vi "Measurement Logic.vi"() -> ()   [LabVIEW 2024, in "NIDmmDCRmsVoltage.lvlib"]
uses:
  NIDmmDCRmsVoltage.lvlib
  <vilib>/MeasurementLink/MeasurementLink Measurement Server/Measure Call Context/Measure Call Context.lvclass
  Typedefs/Measurement Result.ctl
  Typedefs/Measurement Configuration.ctl
  Typedefs/Function.ctl
  Typedefs/Resolution Digits.ctl
  <instrlib>/niDMM/nidmm.llb/niDMM Resolution in Digits.ctl
  <instrlib>/niDMM/nidmm.llb/niDMM Read Waveform (waveform data).vi
  <vilib>/measure/madcrms.llb/Basic Averaged DC-RMS for 1 Chan.vi
  <vilib>/MeasurementLink/MeasurementLink Session Management V1/Session Reservation/Session Reservation.lvclass
  <vilib>/MeasurementLink/MeasurementLink niDMM/MeasurementLink niDMM.lvlib
  <vilib>/MeasurementLink/MeasurementLink niDMM/Initialize Sessions - 1Sess.vi
  <instrlib>/niDMM/nidmm.llb/niDMM Configure Measurement Digits.vi
  <vilib>/measure/NI_MAPro.lvlib
panel:
  in  "measurement configuration":T1={"Range"=10.0, "Function"=1003, "Resolution in Digits"=enum."5 1/2", "Number of Samples"=2000.0, "Pin Name"="", "Sample Rate (Hz)"=20000.0} {"Function" items=["Waveform_Voltage"=1003, "Waveform_Current"=1004]}
  out "Waveform Graph 2":waveform(dbl)(graph)
  in  "Instrument Descriptor":refnum<k15>="DMM1"
  in  "error in":errorcluster
  out "error out":errorcluster
  out "measurement results":T4
  out "measure call context out":refnum<class "Measure Call Context.lvclass">
  in  "measure call context in":refnum<class "Measure Call Context.lvclass">
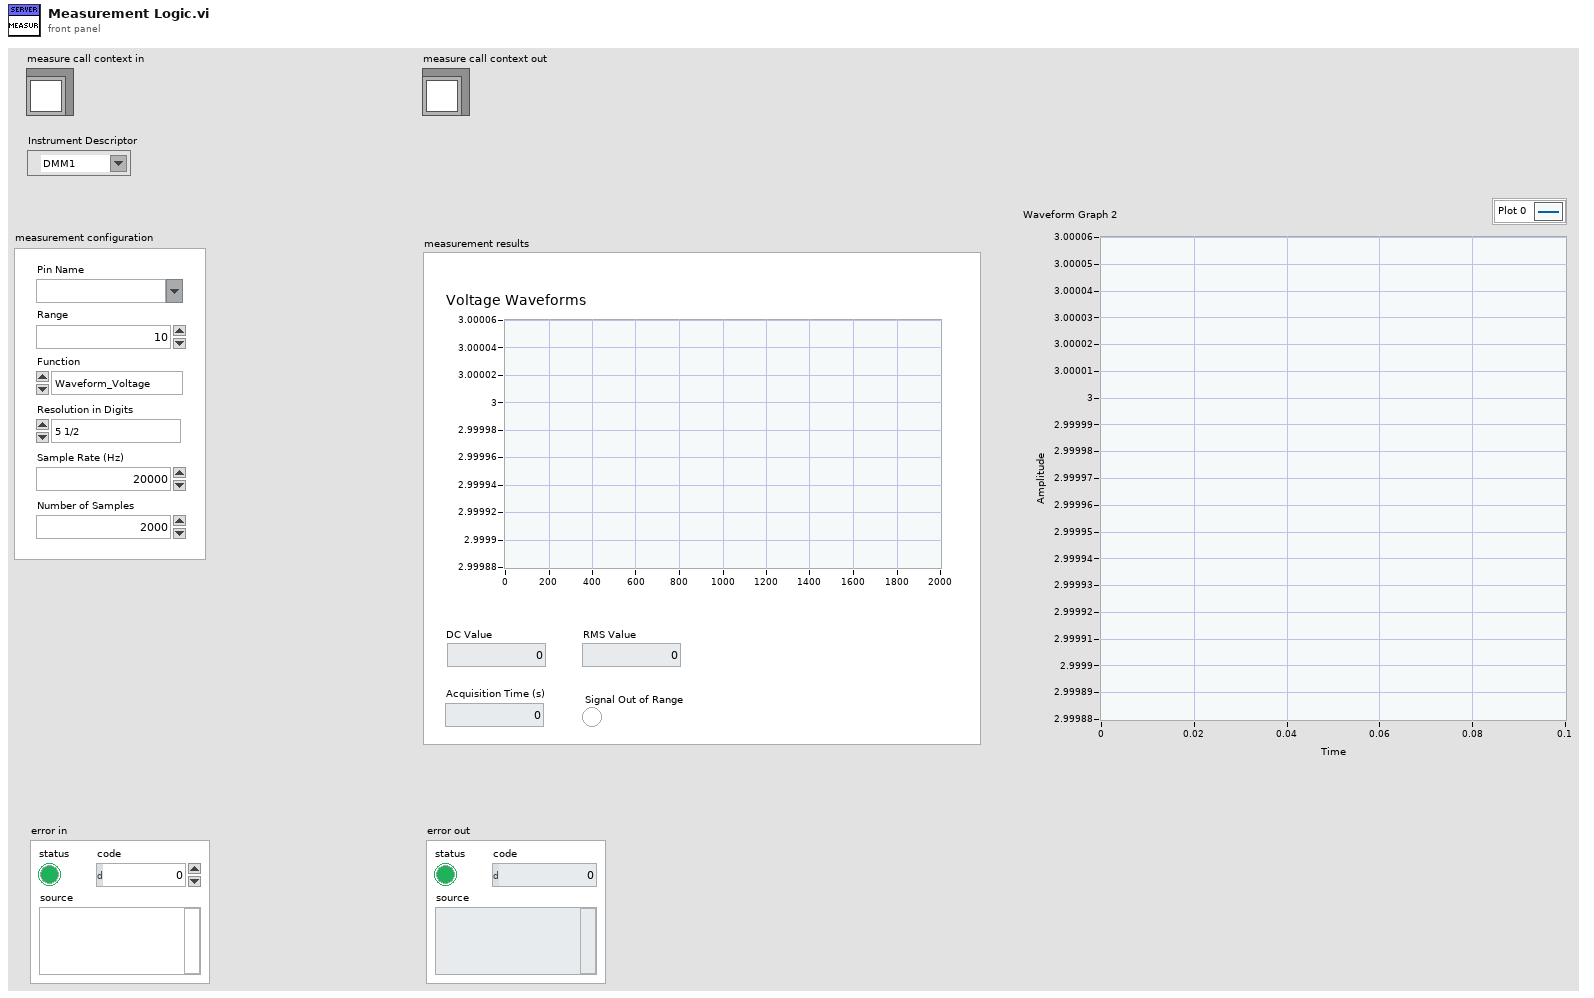
[diagram p1: front panel]
types:
  T1 = typedef "Measurement Configuration.ctl" = cluster{"Range":dbl, "Function":T2, "Resolution in Digits":T3, "Number of Samples":dbl, "Pin Name":string, "Sample Rate (Hz)":dbl}
  T2 = typedef "Function.ctl" = i32
  T3 = typedef "NIDmmDCRmsVoltage.lvlib/Resolution Digits.ctl" = enum32{"3 1/2", "4 1/2", "5 1/2", "6 1/2", "7 1/2"}
  T4 = typedef "NIDmmDCRmsVoltage.lvlib/Measurement Result.ctl" = cluster{"Voltage Waveforms":dbl[], "DC Value":dbl, "RMS Value":dbl, "Acquisition Time (s)":dbl, "Signal Out of Range":bool}
  T5 = typedef "niDMM Resolution in Digits.ctl" = dbl
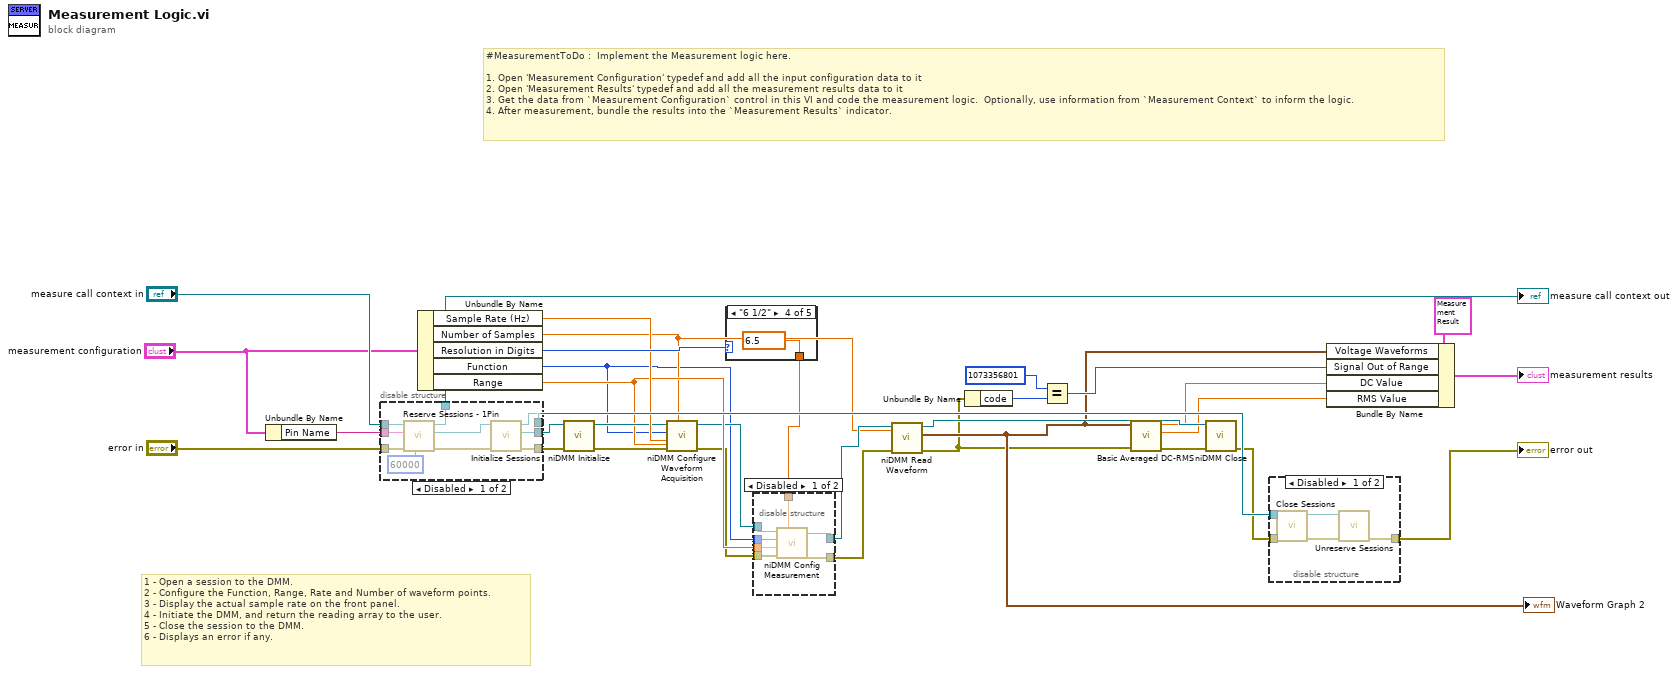
[diagram p0: block diagram]
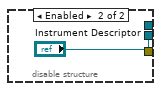
[diagram p4: hidden frame]
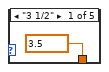
[diagram p5: hidden frame]
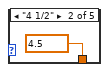
[diagram p6: hidden frame]
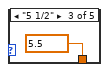
[diagram p7: hidden frame]
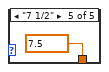
[diagram p8: hidden frame]
diagram:
  # "1 - Open a session to the DMM.\n2 - Configure the Function, Range, Rate and Number of waveform points.\n3 - Display the actual sample rate on the front panel.\n4 - Initiate the DMM, and return the reading array to the user.\n5 - Close the session to the DMM.\n6 - Displays an error if any."
  # "#MeasurementToDo :  Implement the Measurement logic here.\n\n1. Open 'Measurement Configuration' typedef and add all the input configuration data to it\n2. Open 'Measurement Results' typedef and add all the measurement results data to it\n3. Get the data from `Measurement Configuration` control in this VI and code the measurement logic.  Optionally, use information from `Measurement Context` to inform the logic.\n4. After measurement, bundle the results into the `Measurement Results` indicator."
  n1 = Unbundle By Name("measurement configuration") -> ("Pin Name"=w33:string)
  n2 = disable-structure shown="Disabled" {
    disable-tunnel: w33 -> [w43 _]
    disable-tunnel: [w40 _] -> w32
    disable-tunnel: "measure call context in" -> [w38 _]
    disable-tunnel: [w37 _] -> w28
    disable-tunnel: "error in" -> [w36 _]
    disable-tunnel: [w35 "Instrument Descriptor"] -> w24
    disable-tunnel: [w34 _] -> w23
    frame Disabled {
      n3 = call <vilib>:"Reserve Sessions - 1Pin.vi"("timeout (ms)"=60000, "error in"=w36, "pin or relay name"=w43, "measurement context in"=w38) -> ("error out"=w41:errorcluster, "session reservation out"=w42:refnum<class "Session Reservation.lvclass">, "measurement context out"=w37:refnum<class "Measure Call Context.lvclass">)  [unwired: 5 in]
      n4 = call-poly <vilib>:"Initialize Sessions.vi"("error in"=w41, "session reservation in"=w42) -> ("error out"=w34:errorcluster, "session"=w35:refnum<k15>, "session reservation out"=w40:refnum<class "Session Reservation.lvclass">)  [unwired: 6 in, 1 out]
    }
    frame Enabled {
    }
  }
  "measure call context out" <- w28
  n5 = Unbundle By Name("measurement configuration") -> ("Sample Rate (Hz)"=w21:dbl, "Number of Samples"=w9:dbl, "Resolution in Digits"=w31:T3, "Function"=w1:T2, "Range"=w19:dbl)
  n6 = call <instrlib>:"niDMM Initialize.vi"("error in (no error)"=w23, "Instrument Descriptor"=w24) -> ("error out"=w22:errorcluster, "instrument handle out"=w20:refnum<k15>)  [unwired: 8 in]
  n7 = call <instrlib>:"niDMM Configure Waveform Acquisition.vi"("Range"=w19, "Waveform Points"=w9, "error in (no error)"=w22, "Rate"=w21, "Function"=w1, "instrument handle"=w20) -> ("error out"=w18:errorcluster, "instrument handle out"=w17:refnum<k15>)  [unwired: 4 in]
  n8 = case shown="\"6 1/2\"" w31 {
    tunnel: [w45 w46 w47 w48 w49] -> w30
    frame "3 1/2" {
      w45 = T5 3.5 items=["3 1/2"=3.5, "4 1/2"=4.5, "5 1/2"=5.5, "6 1/2"=6.5, "7 1/2"=7.5] ("Resolution in Digits")
    }
    frame "4 1/2" {
      w46 = T5 4.5 items=["3 1/2"=3.5, "4 1/2"=4.5, "5 1/2"=5.5, "6 1/2"=6.5, "7 1/2"=7.5] ("Resolution in Digits")
    }
    frame "5 1/2" {
      w47 = T5 5.5 items=["3 1/2"=3.5, "4 1/2"=4.5, "5 1/2"=5.5, "6 1/2"=6.5, "7 1/2"=7.5] ("Resolution in Digits")
    }
    frame "6 1/2" {
      w48 = T5 6.5 items=["3 1/2"=3.5, "4 1/2"=4.5, "5 1/2"=5.5, "6 1/2"=6.5, "7 1/2"=7.5] ("Resolution in Digits")
    }
    frame "7 1/2" {
      w49 = T5 7.5 items=["3 1/2"=3.5, "4 1/2"=4.5, "5 1/2"=5.5, "6 1/2"=6.5, "7 1/2"=7.5] ("Resolution in Digits")
    }
  }
  n9 = disable-structure shown="Disabled" {
    disable-tunnel: w1 -> [w56 _]
    disable-tunnel: w30 -> [w55 _]
    disable-tunnel: w19 -> [w54 _]
    disable-tunnel: w18 -> [w53 w58]
    disable-tunnel: w17 -> [w52 w57]
    disable-tunnel: [w51 w58] -> w16
    disable-tunnel: [w50 w57] -> w15
    frame Disabled {
      n10 = call-poly <instrlib>:"niDMM Config Measurement.vi"("Range"=w54, "Resolution in Digits"=w55, "error in (no error)"=w53, "Function"=w56, "instrument handle"=w52) -> ("error out"=w51:errorcluster, "instrument handle out"=w50:refnum<k15>)  [unwired: 5 in]
    }
    frame Enabled {
    }
  }
  n11 = call-poly <instrlib>:"niDMM Read Waveform.vi"("Number To Read"=w9, "error in (no error)"=w16, "instrument handle"=w15) -> ("error out"=w7:errorcluster, "Waveform Data"=w8:waveform(dbl), "instrument handle out"=w14:refnum<k15>)  [unwired: 5 in, 1 out]
  "Waveform Graph 2" <- w8
  n12 = Unbundle By Name(w7) -> ("code"=w13:i32)
  n13 = Equal?(x=1073356801 ("y"), y=w13) -> (x = y?=w10:bool)
  n14 = call-poly <vilib>:"Basic Averaged DC-RMS.vi"("error in (no error)"=w7, "signal in"=w8) -> ("error out"=w6:errorcluster, "RMS value"=w3:dbl, "DC value"=w4:dbl)  [unwired: 6 in, 1 out]
  n15 = call <instrlib>:"niDMM Close.vi"("error in (no error)"=w6, "instrument handle"=w14) -> ("error out"=w11:errorcluster)  [unwired: 9 in]
  n16 = disable-structure shown="Disabled" {
    disable-tunnel: w32 -> [w61 _]
    disable-tunnel: [w60 _] -> w26
    disable-tunnel: w11 -> [w59 _]
    frame Disabled {
      n17 = call <vilib>:"Close Sessions.vi"("error in"=w59, "session reservation in"=w61) -> ("error out"=w63:errorcluster, "session reservation out"=w62:refnum<class "Session Reservation.lvclass">)  [unwired: 8 in]
      n18 = call <vilib>:"Unreserve Sessions.vi"("error in"=w63, "session reservation in"=w62) -> ("error out"=w60:errorcluster)  [unwired: 9 in]
    }
    frame Enabled {
    }
  }
  "error out" <- w26
  n19 = Bundle By Name(cluster=T4 {"Voltage Waveforms"=array[2000 elements], "DC Value"=0.0, "RMS Value"=0.0, "Acquisition Time (s)"=0.0, "Signal Out of Range"=FALSE} ("measurement results"), "Voltage Waveforms"=w8, "Signal Out of Range"=w10, "DC Value"=w4, "RMS Value"=w3) -> (→"measurement results":T4)
